vi "Do.vi"(8 "error in (no error)":cluster{"状态":bool, "代码":i32, "源":string} caption="错误输入（无错误）", 10 "操作者输入":refnum<class "Actor.lvclass">, 11 "?":refnum<class "Update Fan Status Msg.lvclass">) -> (0 "error out":cluster{"状态":bool, "代码":i32, "源":string} caption="错误输出", 2 "操作者输出":refnum<class "Actor.lvclass">)   [LabVIEW 2015, in "Evaporative Cooler Controller.lvlib" / "Update Fan Status Msg.lvclass"]
uses:
  Update Fan Status Msg.lvclass
  <vilib>/ActorFramework/Actor/Actor.lvclass
  Evaporative Cooler Controller/Evaporative Cooler Controller.lvclass
  Update Fan Status Msg.lvclass/Update Fan Status Msg.ctl
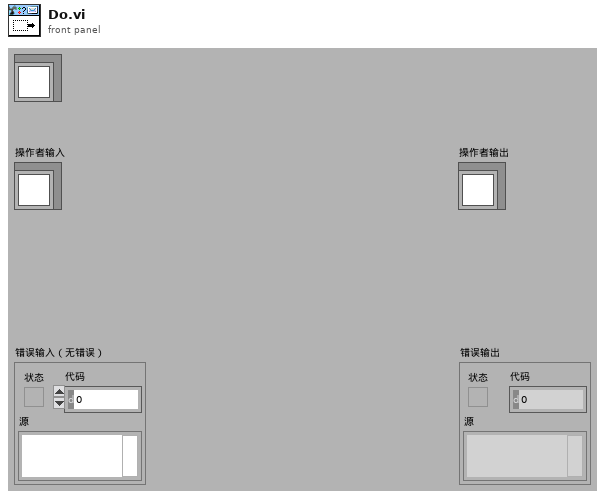
[diagram p1: front panel]
types:
  T1 = typedef "Dual Fan.lvlib/Dual Fan.lvclass/Fan Info.ctl" = cluster{"状态":bool, "故障":bool}
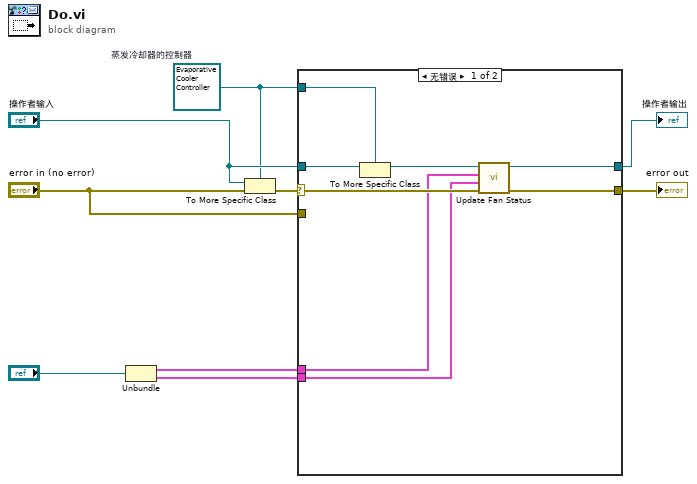
[diagram p0: block diagram]
diagram:
  w4 = refnum<class "Evaporative Cooler Controller.lvclass"> refnum  # 蒸发冷却器的控制器
  n1 = Unbundle("?") -> (w3:T1, w2:T1)
  n2 = To More Specific Class(target class=w4, reference="操作者输入", error in="error in (no error)") -> (error out=w8:errorcluster)  [unwired: 1 out]
  n3 = case shown="无错误" w8 {
    selector: w8 -> [w15 _]
    tunnel: [w17 w18] -> w7
    tunnel: [w16 w19] -> w6
    tunnel: "操作者输入" -> [w14 w19]
    tunnel: w4 -> [w13 _]
    tunnel: w3 -> [w11 _]
    tunnel: w2 -> [w10 _]
    tunnel: "error in (no error)" -> [_ w18]
    frame No Error {
      n4 = To More Specific Class(target class=w13, reference=w14) -> (specific class reference=w12:refnum<class "Evaporative Cooler Controller.lvclass">)  [unwired: 1 in, 1 out]
      n5 = call-dynamic "Update Fan Status.vi"("error in (no error)"=w15, "风扇B"=w10, "风扇A"=w11, "蒸发冷却器的控制器输入"=w12) -> ("error out"=w17:cluster{"状态":bool, "代码":i32, "源":string}, "蒸发冷却器的控制器输出"=w16:refnum<class "Evaporative Cooler Controller.lvclass">)  [unwired: 6 in]
    }
    frame Error {
      # "该Do.vi与标准的Do.vi有点不同。此处如控制器的类型不正确也没有关系。如“转换为特定的类”函数输出错误，直接忽略该错误。这样做的好处是，蒸发冷却器能由普通的“冷却器的控制器”控制，即便普通的“冷却器的控制器” 无法处理蒸发冷却器的所有消息输出。由于输出的都是状态消息，可以不做特殊处理。"
    }
  }
  "error out" <- w7
  "操作者输出" <- w6
